vi "ResonanceAnalyzer.vi"() -> ()   [LabVIEW 2014]
uses:
  <vilib>/imath/engines/lvmath2/RunTimeEngine/Managers/WorkSpace/UID Generator.vi
  <vilib>/imath/engines/lvmath2/RunTimeEngine/RangeToken/NIMS_Range.vi
  <instcachedir>/0/NIMS_Range_9BCE657718DF4976A877346C61F22738.lvgen/NIMS_Range_9BCE657718DF4976A877346C61F22738_000.vi
  <vilib>/imath/engines/lvmath2/RunTimeEngine/RunTimeType/NIMS_RunTimeType_From StrictType (excl LVString).vi
  <instcachedir>/0/NIMS_RunTimeType_From StrictType (excl LVString)_15A5391EEA9C4AACB9955AC755B83D29.lvgen/NIMS_RunTimeType_From StrictType (excl LVString)_15A5391EEA9C4AACB9955AC755B83D29_000.vi
  <vilib>/imathl/engines/lvmath/Functions/Error Handling/Create Error.vi
  <vilib>/imath/engines/lvmath2/RunTimeEngine/LocalVariableDefStatement/MC_LocalVariableDefStatement_Display.vi
  <vilib>/imath/engines/lvmath2/RunTimeEngine/ArithmeticOperatorToken/NIMS_ArithmeticOperator_minus.vi
  <instcachedir>/0/NIMS_ArithmeticOperator_minus_39C0593E74DA4138ACA2AB742906488D.lvgen/NIMS_ArithmeticOperator_minus_39C0593E74DA4138ACA2AB742906488D_003.vi
  <vilib>/imath/engines/lvmath2/RunTimeEngine/BuiltInFunctions/length/NIMS_length(GV).vi
  <instcachedir>/0/NIMS_length(GV)_08A3D13377FD4E4B96F5795FBF3698FA.lvgen/NIMS_length(GV)_08A3D13377FD4E4B96F5795FBF3698FA_001.vi
  <vilib>/imath/engines/lvmath2/RunTimeEngine/BuiltInFunctions/rand/NIMS_rand(1,I32).vi
  <vilib>/imath/engines/lvmath2/RunTimeEngine/ErrorHandling/NIMS_Error From Error Code.vi
  <vilib>/imath/engines/lvmath2/RunTimeEngine/IndexRead/NIMS M(S,$).vi
  <instcachedir>/0/NIMS M(S,$)_F24F360562DE41D8BE234322A2E15C65.lvgen/NIMS M(S,$)_F24F360562DE41D8BE234322A2E15C65_001.vi
  <instcachedir>/0/NIMS M(S,$)_F24F360562DE41D8BE234322A2E15C65.lvgen/NIMS M(S,$)_F24F360562DE41D8BE234322A2E15C65_000.vi
  <vilib>/imath/engines/lvmath2/RunTimeEngine/ArithmeticOperatorToken/NIMS_ArithmeticOperator_plus.vi
  <instcachedir>/0/NIMS_ArithmeticOperator_plus_48D6EAACA5D645B09F7EC9C016C2DEA8.lvgen/NIMS_ArithmeticOperator_plus_48D6EAACA5D645B09F7EC9C016C2DEA8_000.vi
  <vilib>/imath/engines/lvmath2/RunTimeEngine/ErrorHandling/NIMS_Create Error From Enums.vi
  <vilib>/imath/engines/lvmath2/RunTimeEngine/Managers/SymbolTable/Clear UID.vi
  <vilib>/imath/engines/lvmath2/RunTimeEngine/NodeEndStatement/NIMS_NodeEndStatement_Output.vi
  <instcachedir>/0/NIMS_NodeEndStatement_Output_53EC0D466D134D7ABD903AC30B43404B.lvgen/NIMS_NodeEndStatement_Output_53EC0D466D134D7ABD903AC30B43404B_005.vi
  <instcachedir>/0/NIMS_NodeEndStatement_Output_53EC0D466D134D7ABD903AC30B43404B.lvgen/NIMS_NodeEndStatement_Output_53EC0D466D134D7ABD903AC30B43404B_000.vi
  <vilib>/imath/engines/lvmath2/RunTimeEngine/ErrorHandling/NIMS_Finalize Error.vi
  <vilib>/imath/engines/lvmath2/RunTimeEngine/Managers/SymbolTable/NIMS_WorkSpace.lvlib
panel:
  out "Output Cluster":T1
  out "XY Graph":cluster{"out":dbl[], "freq":dbl[]}[](graph)
  in  "Tab Control":enum32{"SImulation", "Experiment"}(tab)
  in  "Input Parameters":T2
  in  "Filename":path
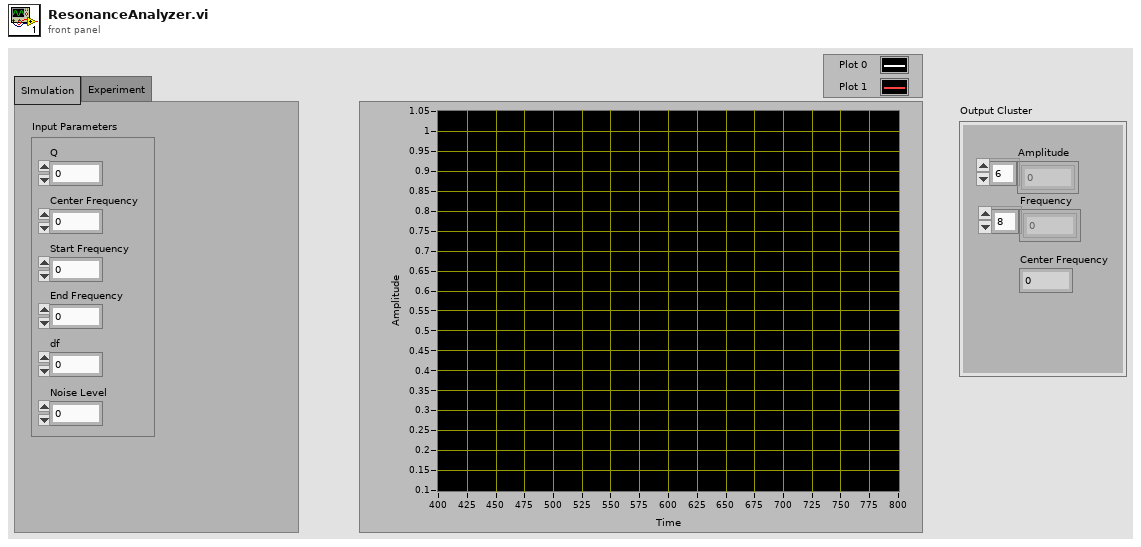
[diagram p1: front panel]
types:
  T1 = cluster{"Amplitude":cdb[], "Frequency":dbl[], "Center Frequency":dbl}
  T2 = cluster{"Q":dbl, "Center Frequency":dbl, "Start Frequency":dbl, "End Frequency":dbl, "df":dbl, "Noise Level":dbl}
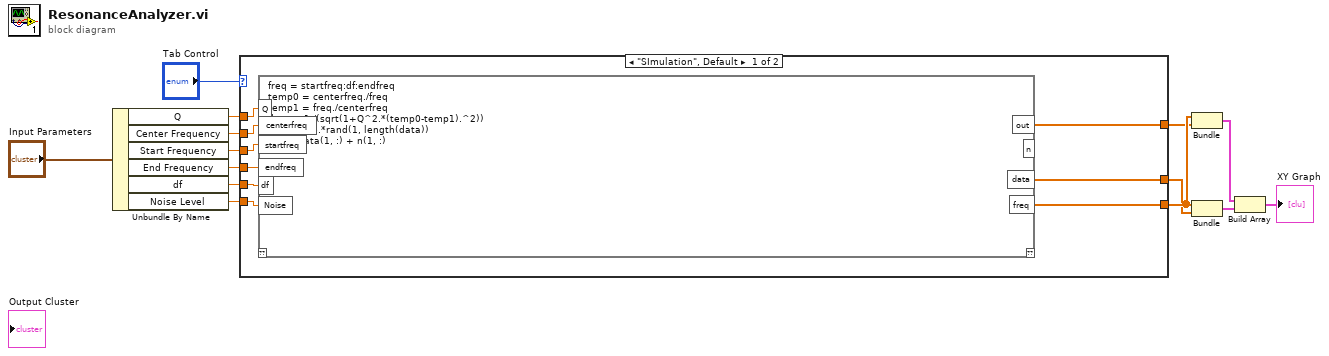
[diagram p0: block diagram]
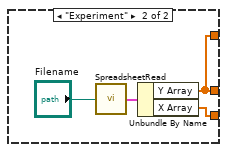
[diagram p2: hidden frame]
diagram:
  n1 = Unbundle By Name("Input Parameters") -> ("Q"=w10:dbl, "Center Frequency"=w9:dbl, "Start Frequency"=w8:dbl, "End Frequency"=w7:dbl, "df"=w6:dbl, "Noise Level"=w5:dbl)
  n2 = case shown="\"SImulation\", Default" "Tab Control" {
    tunnel: [w15 w218] -> w2
    tunnel: [w22 w220] -> w4
    tunnel: w10 -> [w21 _]
    tunnel: w9 -> [w20 _]
    tunnel: w8 -> [w19 _]
    tunnel: w7 -> [w18 _]
    tunnel: w6 -> [w17 _]
    tunnel: w5 -> [w16 _]
    tunnel: [w23 w218] -> w3
    frame "SImulation", Default {
      n3 = mathscript code="freq = startfreq:df:endfreq\ntemp0 = centerfreq./freq\ntemp1 = freq./centerfreq\ndata = 1./(sqrt(1+Q^2.*(temp0-temp1).^2))\nn =  Noise.*rand(1, length(data))\nout = data(1, :) + n(1, :)"("Q"=w21, "centerfreq"=w20, "startfreq"=w19, "endfreq"=w18, "df"=w17, "Noise"=w16) -> ("out"=w15:cdb[], "data"=w23:cdb[], "freq"=w22:dbl[])  [unwired: 1 in, 2 out]
    }
    frame "Experiment" {
      n4 = call "SpreadsheetRead.vi"("Path"="Filename") -> ("Output Cluster"=w221:cluster{"Y Array":dbl[], "X Array":dbl[]})
      n5 = Unbundle By Name(w221) -> ("Y Array"=w218:dbl[], "X Array"=w220:dbl[])
    }
  }
  n6 = Bundle("X Array"=w4, "out"=w2) -> (w13:cluster{"X Array":dbl[], "out":cdb[]})  [unwired: 1 in]
  n7 = Bundle("X Array"=w4, "data"=w3) -> (w12:cluster{"X Array":dbl[], "data":cdb[]})  [unwired: 1 in]
  n8 = Build Array(w13, w12) -> (→"XY Graph":cluster{"X Array":dbl[], "data":cdb[]}[])
